vi "Limelight Controller.vi"(8 "error in":errorcluster) -> ()   [LabVIEW 2018]
doc: "This VI executes continuously carrying out the current operation and responding to updates or new operations. It will often contain the timing or control code that is difficult to place directly in TeleOp. This VI generally opens all sensors and motors and isolates the rest of the robot code from knowing how the operations are carried out."
uses:
  <vilib>/Rock Robotics/WPI/Framework/Completion Status.ctl
  Limelight Setpoints.ctl
  Limelight Operations.ctl
  Pipeline Index.ctl
  <vilib>/Rock Robotics/Network Tables/NT Read Number.vi
  Limelight Published Globals.vi
  <vilib>/Rock Robotics/Network Tables/NT Write Boolean.vi
  <vilib>/Rock Robotics/Network Tables/NT Write Number.vi
panel:
  in  "Interactive Values":T1
  out "Current\nCmd":string
  in  "Buttons":cluster{"Execute Cmd":bool, "Abort Cmd":bool}
  out "Command Timing":cluster{"Start Time (ms)":u32, "Iterations":i32}
  out "Status":T3
  # "Tip: It may be helpful to observe inputs and sensor values.\nYou may also want to display tuning or debugging controls."
  # "Interactive Command: You may fill in the settings for a command\nand schedule it with the Execute button. You can observe and abort\nany command while fine tuning the code for the controller."
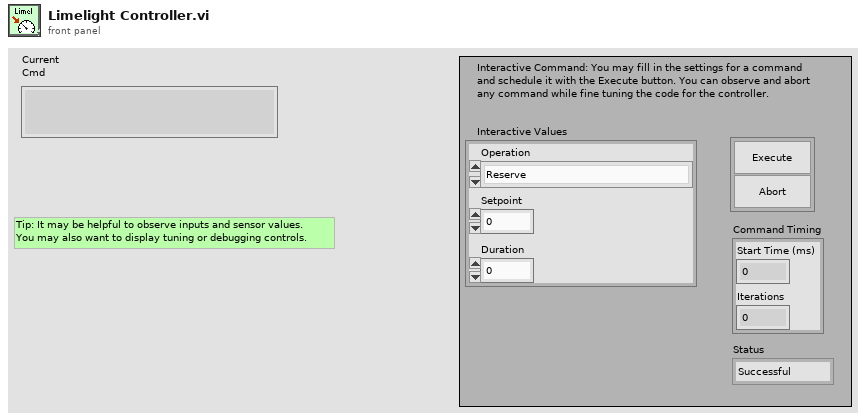
[diagram p1: front panel]
types:
  T1 = typedef "Limelight Setpoints.ctl" = cluster{"Operation":T2, "Setpoint":dbl, "Duration":dbl}
  T2 = typedef "Limelight Operations.ctl" = enum16{"Reserve", "Read Current", "Immediate", "Pipeline Change"}
  T3 = typedef "Completion Status.ctl" = enum16{"Successful", "Aborted", "Incomplete"}
  T4 = typedef "Command Status Info.ctl" = cluster{"Name":string, "Status":T3, "notifier out":T5}
  T5 = typedef "Completion Notifier.ctl" = refnum<notifier>
  T6 = cluster{"Current Command":T1, "Command Timing":cluster{"Start Time (ms)":u32, "Iterations":i32}, "Command Arguments":cluster{"Command Info":T4, "Description":string, "Default Command":T1, "queue out":refnum<queue>, "Subsystem Name":string}}
  T7 = typedef "Pipeline Index.ctl" = enum16{"Cargo", "Hatch", "Vision"}
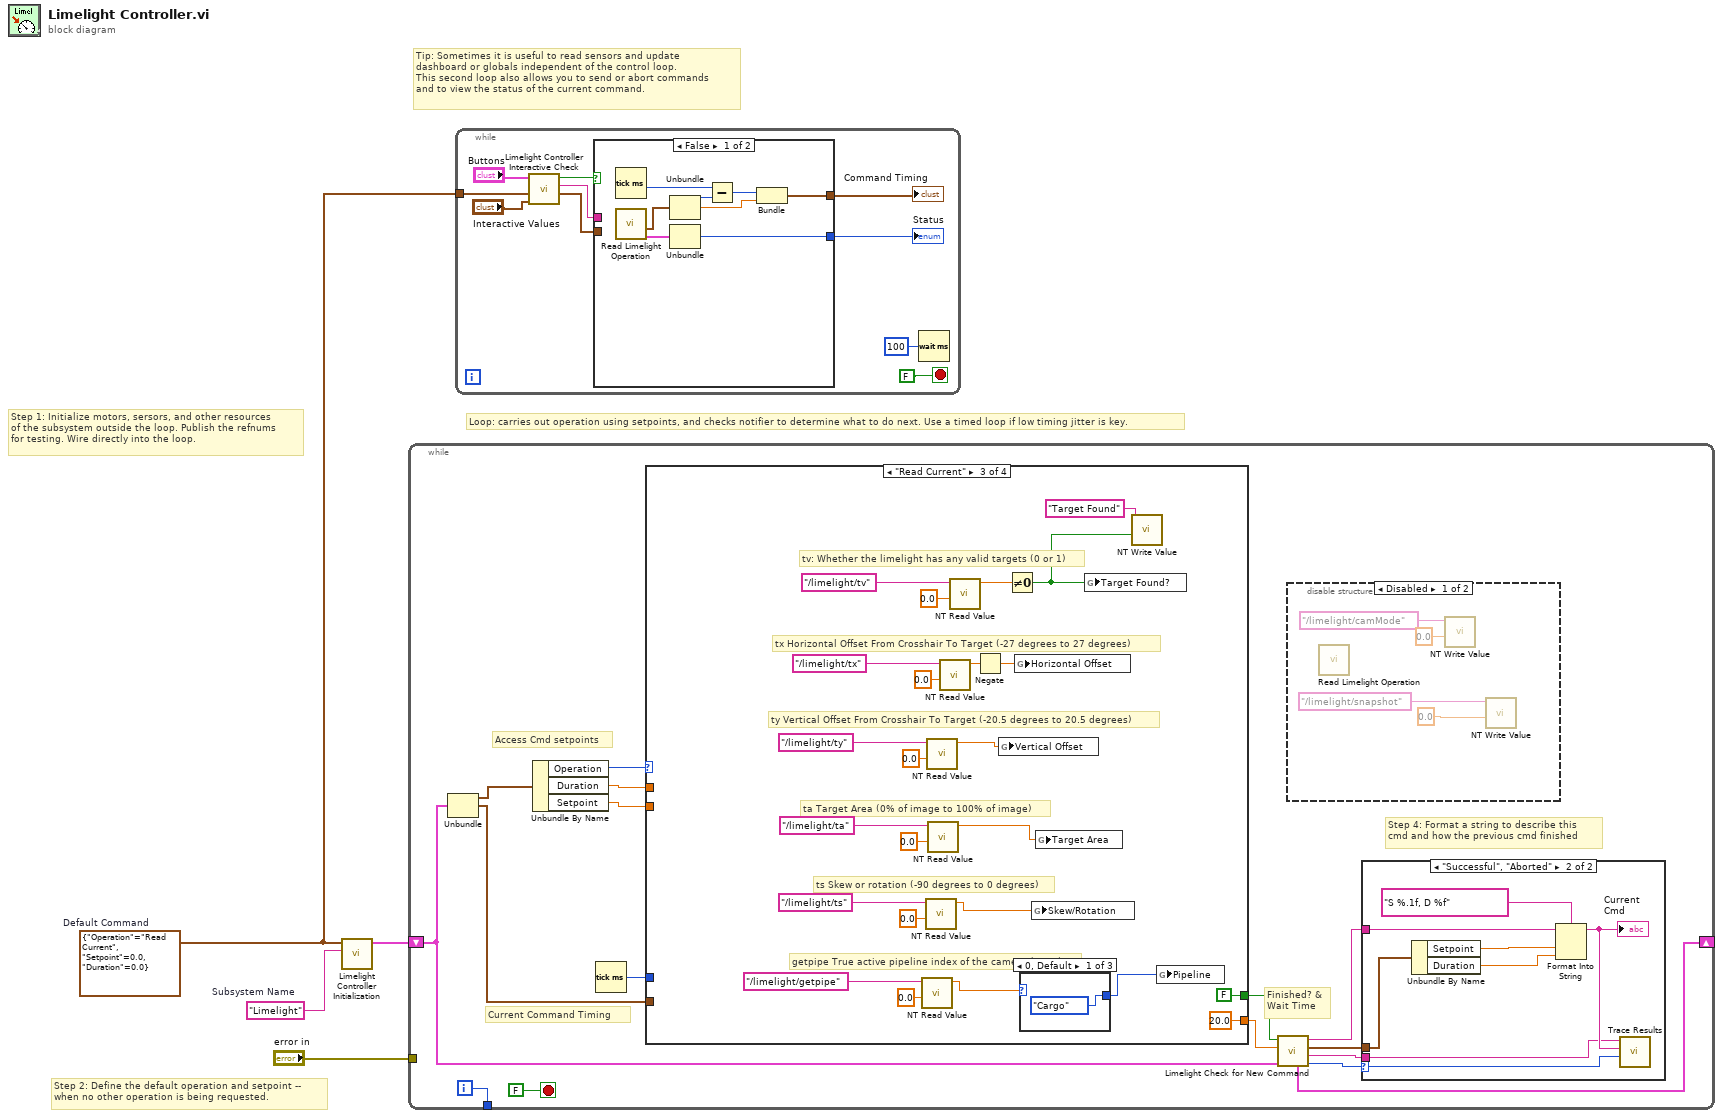
[diagram p0: block diagram]
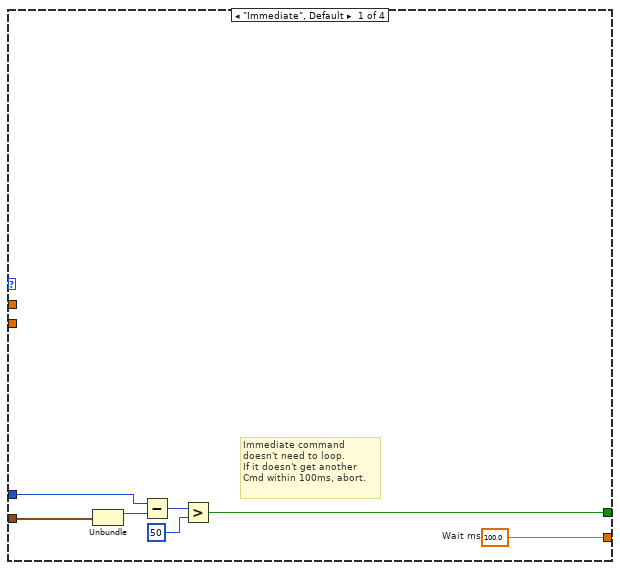
[diagram p4: hidden frame]
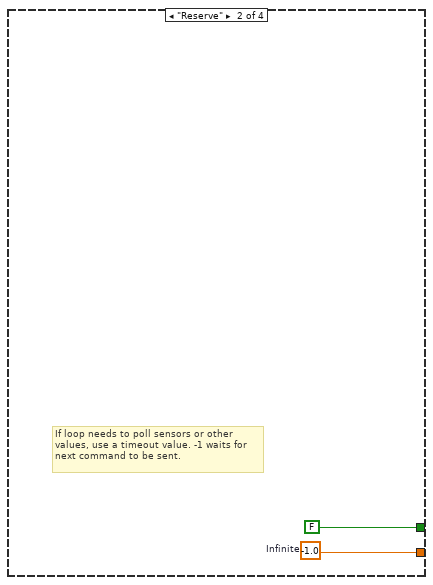
[diagram p5: hidden frame]
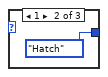
[diagram p6: hidden frame]
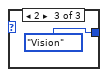
[diagram p7: hidden frame]
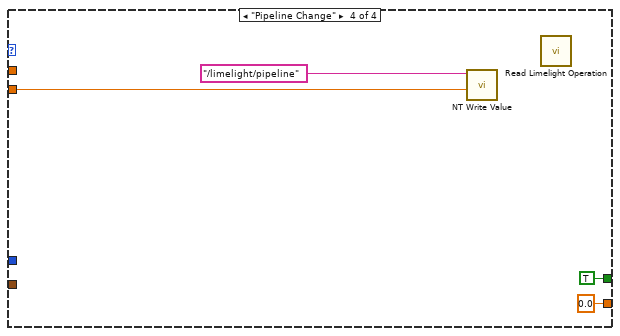
[diagram p8: hidden frame]
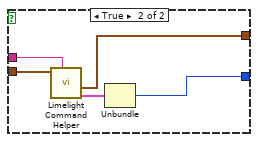
[diagram p9: hidden frame]
diagram:
  w1 = T1 {"Operation"=enum."Read Current", "Setpoint"=0.0, "Duration"=0.0}  # Default Command
  w2 = "Limelight"  # Subsystem Name
  # "Tip: Sometimes it is useful to read sensors and update\ndashboard or globals independent of the control loop.\nThis second loop also allows you to send or abort commands\nand to view the status of the current command."
  # "Step 2: Define the default operation and setpoint --\nwhen no other operation is being requested."
  # "Step 1: Initialize motors, sersors, and other resources\nof the subsystem outside the loop. Publish the refnums\nfor testing. Wire directly into the loop."
  # "Loop: carries out operation using setpoints, and checks notifier to determine what to do next. Use a timed loop if low timing jitter is key."
  n1 = call "Limelight Controller Initialization.vi"("Subsystem Name"=w2, "Default Command"=w1) -> ("Current Command"=w3:T6)  [unwired: 9 in]
  n2 = while {
    shift-right: [w12] -> _
    shift-left: w3 -> [w5]
    tunnel: [w19] -> _
    tunnel: "error in" -> [_]
    i -> [w19]
    stop <- FALSE stop-if-true
    # "Step 4: Format a string to describe this\ncmd and how the previous cmd finished"
    # "Current Command Timing"
    # "Access Cmd setpoints"
    # "Finished? &\nWait Time"
    n3 = Unbundle(w5) -> ("Current Command"=w18:T1, "Command Timing"=w14:cluster{"Start Time (ms)":u32, "Iterations":i32})  [unwired: 1 out]
    n4 = Unbundle By Name(w18) -> ("Operation"=w17:T2, "Duration"=w16:dbl, "Setpoint"=w13:dbl)
    n5 = Tick Count (ms)() -> (millisecond timer value=w15:u32)
    n6 = case shown="\"Read Current\"" w17 {
      tunnel: [w39 w41 20.0 ("Infinite") 0.0 ("Infinite")] -> w10
      tunnel: [w33 FALSE ("ignore previous (F)") FALSE ("ignore previous (F)") TRUE ("ignore previous (F)")] -> w11
      tunnel: w14 -> [w35 _ _ _]
      tunnel: w16 -> [_ _ _ _]
      tunnel: w15 -> [w34 _ _ _]
      tunnel: w13 -> [_ _ _ w71]
      frame "Immediate", Default {
        w39 = 100.0  # Wait ms
        # "Immediate command\ndoesn't need to loop.\nIf it doesn't get another\nCmd within 100ms, abort."
        n7 = Unbundle(w35) -> ("Start Time (ms)"=w38:u32)  [unwired: 1 out]
        n8 = Subtract(x=w34, y=w38) -> (x-y=w37:u32)
        n9 = Greater?(x=w37, y=u8 50 ("Left Motor")) -> (0:w33:bool)
      }
      frame "Reserve" {
        w41 = -1.0  # Infinite
        # "If loop needs to poll sensors or other\nvalues, use a timeout value. -1 waits for\nnext command to be sent."
      }
      frame "Read Current" {
        # "getpipe\tTrue active pipeline index of the camera (0 .. 9)"
        # "ts\tSkew or rotation (-90 degrees to 0 degrees)"
        # "ta\tTarget Area (0% of image to 100% of image)"
        # "ty\tVertical Offset From Crosshair To Target (-20.5 degrees to 20.5 degrees)"
        # "tx\tHorizontal Offset From Crosshair To Target (-27 degrees to 27 degrees)"
        # "tv:\tWhether the limelight has any valid targets (0 or 1)"
        n10 = call-poly <vilib>:"NT Read Value.vi"("Default Value"=0.0, "Name"="/limelight/getpipe") -> ("Numeric"=w50:dbl)  [unwired: 8 in, 1 out]
        n11 = call-poly <vilib>:"NT Read Value.vi"("Default Value"=0.0, "Name"="/limelight/ts") -> ("Numeric"=w45:dbl)  [unwired: 8 in, 1 out]
        n12 = call-poly <vilib>:"NT Read Value.vi"("Default Value"=0.0, "Name"="/limelight/ty") -> ("Numeric"=w47:dbl)  [unwired: 8 in, 1 out]
        n13 = call-poly <vilib>:"NT Read Value.vi"("Default Value"=0.0, "Name"="/limelight/ta") -> ("Numeric"=w46:dbl)  [unwired: 8 in, 1 out]
        n14 = call-poly <vilib>:"NT Read Value.vi"("Default Value"=0.0, "Name"="/limelight/tx") -> ("Numeric"=w48:dbl)  [unwired: 8 in, 1 out]
        n15 = call-poly <vilib>:"NT Read Value.vi"("Default Value"=0.0, "Name"="/limelight/tv") -> ("Numeric"=w51:dbl)  [unwired: 8 in, 1 out]
        n16 = Negate(x=w48) -> (-x=w44:dbl)
        n17 = global write "Limelight Published Globals.vi" "Vertical Offset"(w47) -> ()
        n18 = Not Equal To 0?(x=w51) -> (x != 0?=w42:bool)
        n19 = global write "Limelight Published Globals.vi" "Horizontal Offset"(w44) -> ()
        n20 = case shown="0, Default" w50 {
          tunnel: [Pipeline_Index."Cargo" ("Pipeline") Pipeline_Index."Hatch" ("Pipeline") Pipeline_Index."Vision" ("Pipeline")] -> w49
          frame 0, Default {
          }
          frame 1 {
          }
          frame 2 {
          }
        }
        n21 = global write "Limelight Published Globals.vi" "Skew/Rotation"(w45) -> ()
        n22 = global write "Limelight Published Globals.vi" "Target Area"(w46) -> ()
        n23 = global write "Limelight Published Globals.vi" "Target Found?"(w42) -> ()
        n24 = call-poly <vilib>:"NT Write Value.vi"("Boolean"=w42, "Name"="Target Found") -> ()  [unwired: 9 in, 1 out]
        n25 = global write "Limelight Published Globals.vi" "Pipeline"(w49) -> ()
      }
      frame "Pipeline Change" {
        n26 = call-poly <vilib>:"NT Write Value.vi"("Numeric"=w71, "Name"="/limelight/pipeline") -> ()  [unwired: 9 in, 1 out]
        n27 = call "Read Limelight Operation.vi"() -> ()  [unwired: 9 in, 3 out]
      }
    }
    n28 = call "Limelight Check for New Command.vi"("Current Command"=w5, "Wait time (ms)"=w10, "Finished?"=w11) -> ("Completion"=w6:T3, "Subsystem Name"=w7:string, "Current Command"=w8:T1, "Initial Trace String"=w9:string, "NextCommand"=w12:T6)  [unwired: 4 in]
    n29 = disable-structure shown="Disabled" {
      frame Disabled {
        n30 = call "Read Limelight Operation.vi"() -> ()  [unwired: 9 in, 3 out]
        n31 = call-poly <vilib>:"NT Write Value.vi"("Numeric"=0.0 ("Default Value"), "Name"="/limelight/camMode") -> ()  [unwired: 9 in, 1 out]
        n32 = call-poly <vilib>:"NT Write Value.vi"("Numeric"=0.0 ("Default Value"), "Name"="/limelight/snapshot") -> ()  [unwired: 9 in, 1 out]
      }
      frame Enabled {
      }
    }
    n33 = case shown="\"Successful\", \"Aborted\"" w6 {
      selector: w6 -> [_ w32]
      tunnel: w9 -> [_ w28]
      tunnel: w8 -> [_ w29]
      tunnel: w7 -> [_ w25]
      frame "Incomplete", Default {
        # "Continuing current command"
      }
      frame "Successful", "Aborted" {
        # "Report and setup for next command"
        n34 = Unbundle By Name(w29) -> ("Setpoint"=w31:dbl, "Duration"=w26:dbl)
        n35 = Format Into String(format string="S %.1f, D %f", initial string=w28, w31, w26) -> (resulting string=w27:string)  [unwired: 1 in, 1 out]
        "Current\nCmd" <- w27
        n36 = call <vilib>:"Trace Results.vi"("Status of previous command"=w32, "Description"=w27, "Subsystem"=w25) -> ()  [unwired: 9 in]
      }
    }
  }
  n37 = while {
    tunnel: w1 -> [w79]
    stop <- FALSE stop-if-true
    n38 = call "Limelight Controller Interactive Check.vi"("Interactive Command in"="Interactive Values", "Default Command"=w79, "Buttons"="Buttons") -> ("Interactive Command out"=w76:T1, "Trace String"=w77:string, "Schedule"=w78:bool)  [unwired: 6 in]
    n39 = case shown="False" w78 {
      tunnel: [w90 w95] -> w75
      tunnel: w76 -> [_ w93]
      tunnel: [w86 w91] -> w74
      tunnel: w77 -> [_ w94]
      frame False {
        n40 = Tick Count (ms)() -> (millisecond timer value=w85:u32)
        n41 = call "Read Limelight Operation.vi"() -> ("Command Info"=w83:T4, "SubSystem Data"=w84:T1)  [unwired: 9 in, 1 out]
        n42 = Unbundle(w84) -> ("Operation"=w89:T2, "Setpoint"=w87:dbl)  [unwired: 1 out]
        n43 = Unbundle(w83) -> ("Status"=w90:T3)  [unwired: 2 out]
        n44 = Subtract(x=w85, y=w89) -> (x-y=w88:u32)
        n45 = Bundle(w88, "Setpoint"=w87) -> (w86:cluster{u32, "Setpoint":dbl})  [unwired: 1 in]
      }
      frame True {
        n46 = call "Limelight Command Helper.vi"("Description"=w94, "SubSystem Data"=w93) -> ("Command Info Out"=w92:T4, "Command Timing"=w91:cluster{"Start Time (ms)":u32, "Iterations":i32})  [unwired: 7 in, 1 out]
        n47 = Unbundle(w92) -> ("Status"=w95:T3)  [unwired: 2 out]
      }
    }
    "Status" <- w75
    "Command Timing" <- w74
    n48 = Wait (ms)(milliseconds to wait=u32 100) -> ()  [unwired: 1 out]
  }
